vi "Automation Message Loop.vi"(8 "error in (no error)":errorcluster, 10 "Data Notifiers":T1, 11 "Message Queues":T2) -> (0 "error out":errorcluster)   [LabVIEW 2013, in "Automation.lvlib"]
uses:
  Automation.lvlib
  support/Message Queue/All Message Queues.ctl
  support/Message Queue/Message Cluster.ctl
  support/Data Notifiers/All Data Notifiers.ctl
  Acquisition/APD Notifier Cluster.ctl
  Piezo/Piezo display.ctl
  XY/XY Display.ctl
  Capacitive/Capacitive Signal Cluster.ctl
  Feedback/Error Signal.ctl
  Automation State.ctl
  Zscan Settings.ctl
  support/Message Queue/Enqueue Message (Single).vi
  <vilib>/Utility/error.llb/Error Cluster From Error Code.vi
  <vilib>/ErrorRing/Error Ring.xnode
  Piezo/Piezo.lvlib
  support/Message Queue/Message Queue.lvlib
  Acquisition/Acquisition.lvlib
  XY/XY.lvlib
  Capacitive/Capacitive.lvlib
  Feedback/Feedback.lvlib
  support/Data Notifiers/Data Notifiers.lvlib
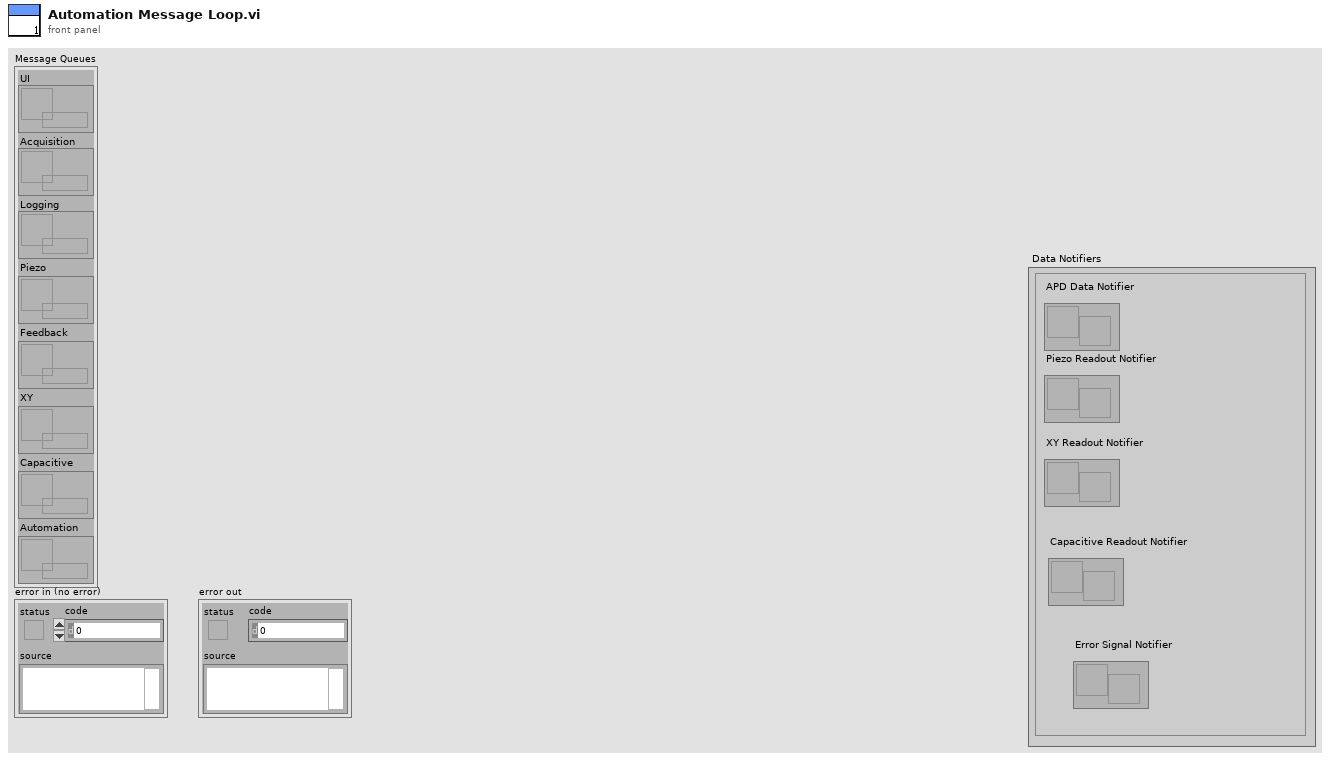
[diagram p1: front panel]
types:
  T1 = typedef "Data Notifiers.lvlib/All Data Notifiers.ctl" = cluster{"APD Data Notifier":refnum<notifier>, "Piezo Readout Notifier":refnum<notifier>, "XY Readout Notifier":refnum<notifier>, "Capacitive Readout Notifier":refnum<notifier>, "Error Signal Notifier":refnum<notifier>}
  T2 = typedef "Message Queue.lvlib/All Message Queues.ctl" = cluster{"UI":refnum<queue>, "Acquisition":refnum<queue>, "Logging":refnum<queue>, "Piezo":refnum<queue>, "Feedback":refnum<queue>, "XY":refnum<queue>, "Capacitive":refnum<queue>, "Automation":refnum<queue>}
  T3 = enum16{"Idle", "Waiting for lock", "Waiting for acquisition"}
  T4 = typedef "Automation.lvlib/Zscan Settings.ctl" = cluster{"Heights":dbl[], "Seconds per height":i32, "First Data Index":i32}
  T5 = typedef "Automation.lvlib/Automation State.ctl" = cluster{"State":enum16{"Idle", "Zscan"}, "Logging?":bool, "Zscan State":cluster{"State":enum16{"Idle", "Waiting for lock", "Waiting for acquisition"}, "ZScan Settings":T4, "Current Step":i32, "Current Cap Height":dbl, "Total Steps":i32, "Time Logging Started":dbl}}
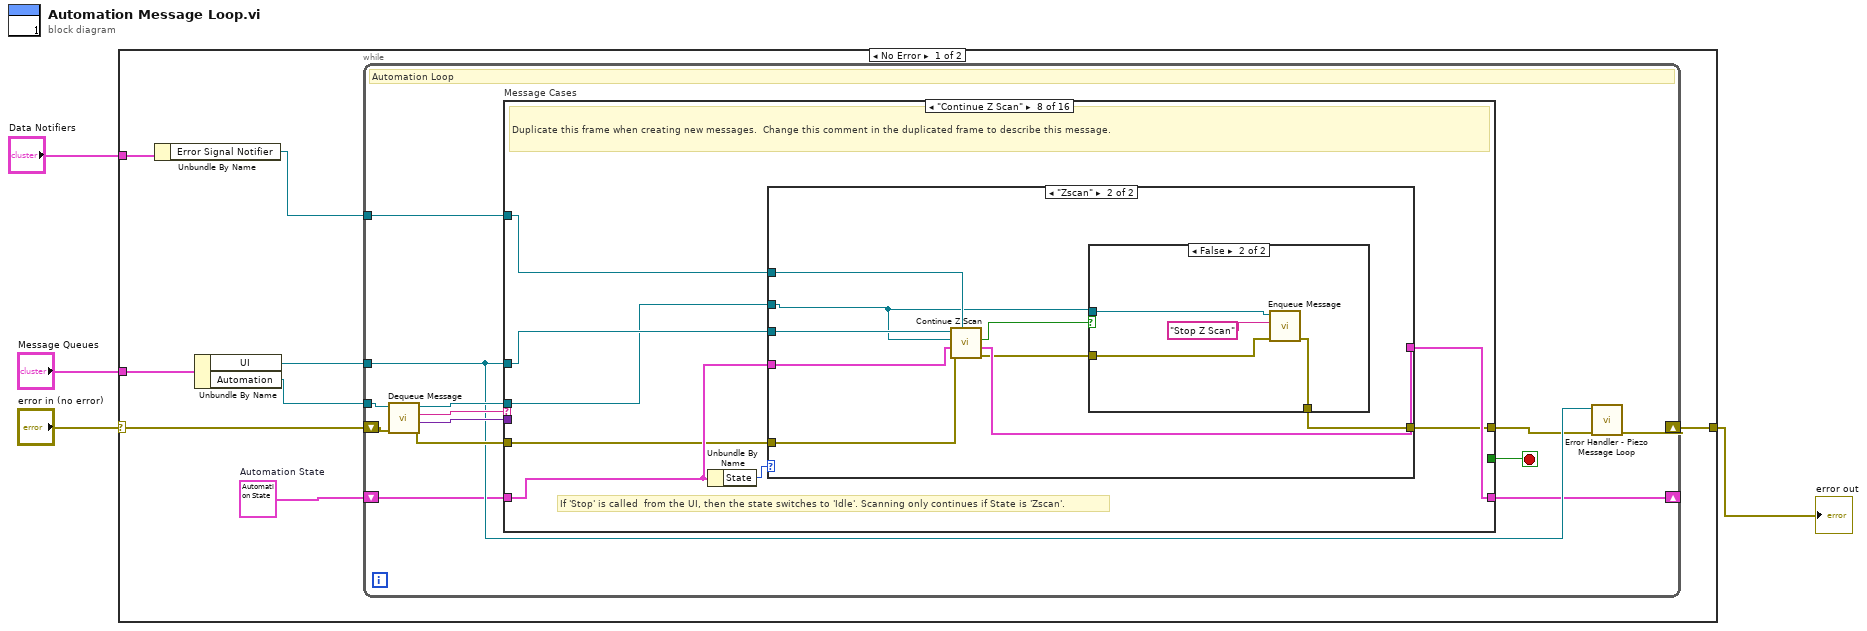
[diagram p0: block diagram]
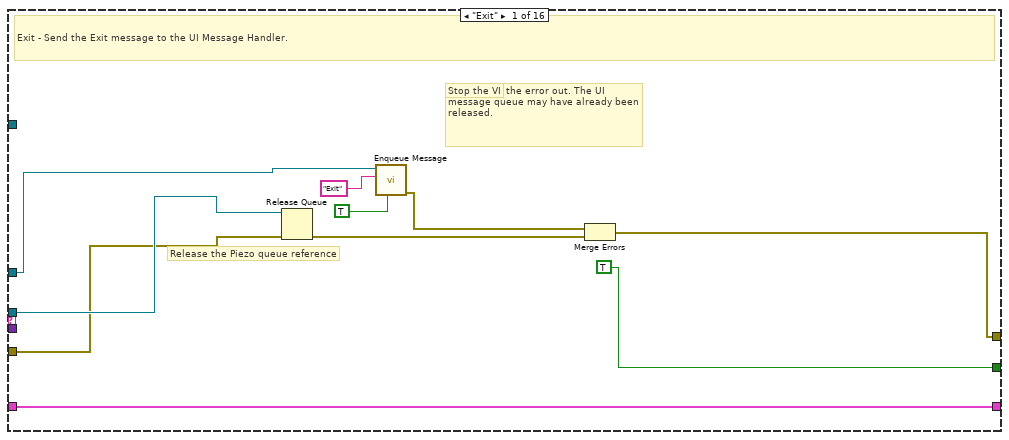
[diagram p2: hidden frame]
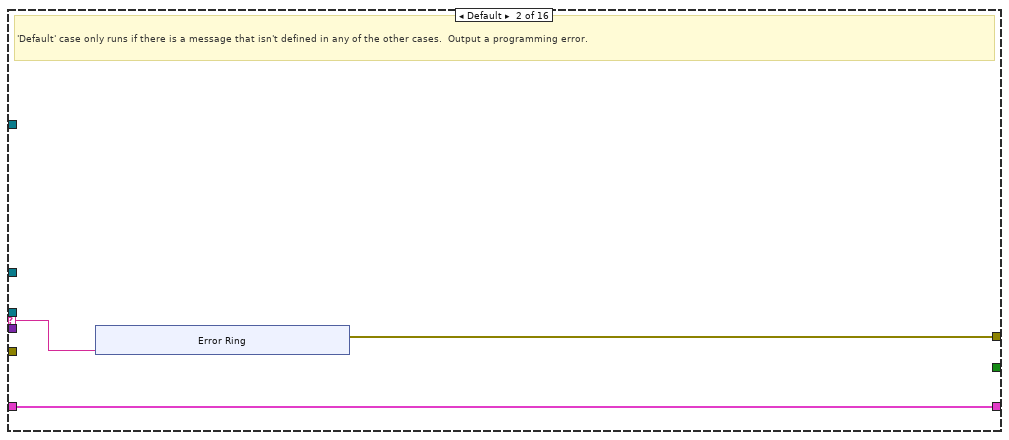
[diagram p3: hidden frame]
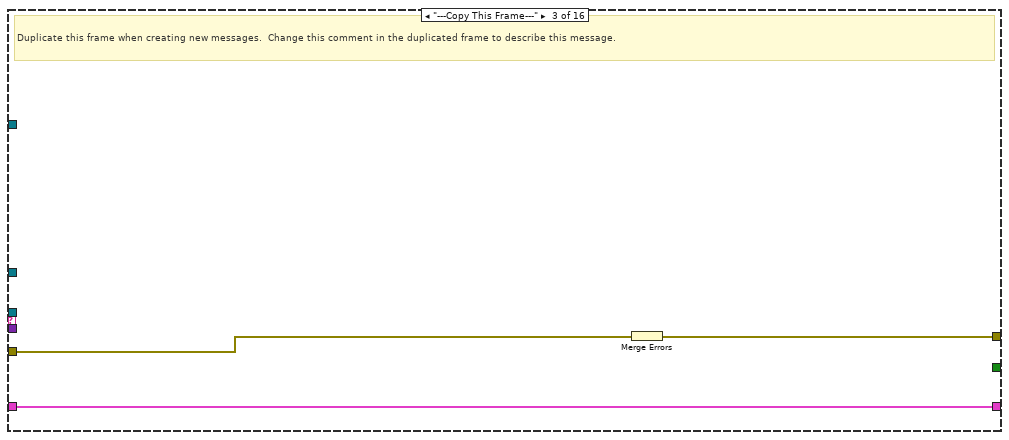
[diagram p4: hidden frame]
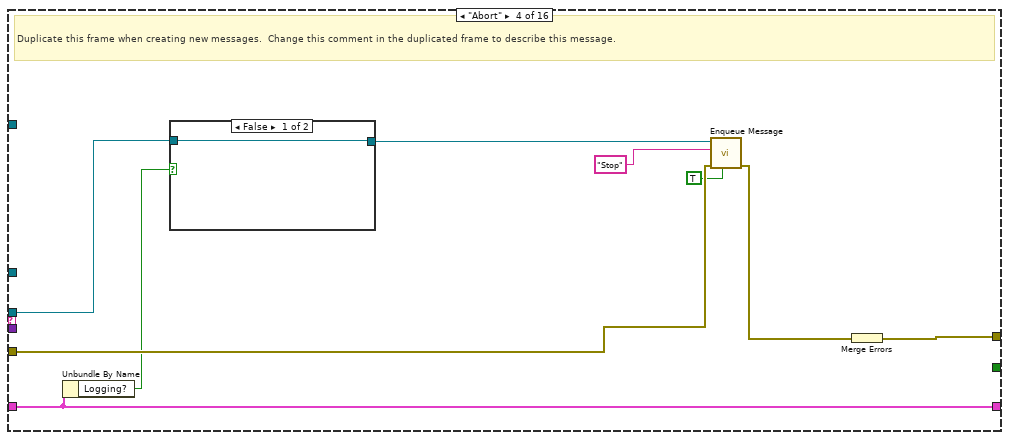
[diagram p5: hidden frame]
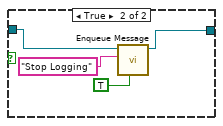
[diagram p6: hidden frame]
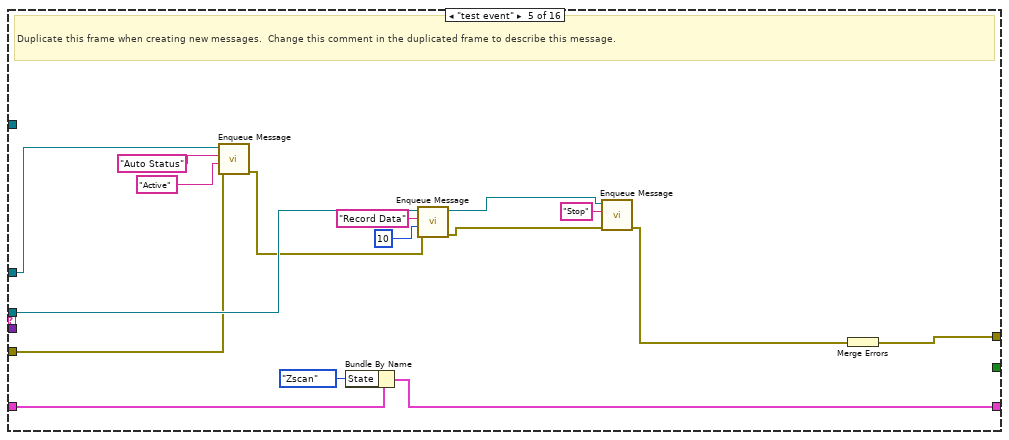
[diagram p7: hidden frame]
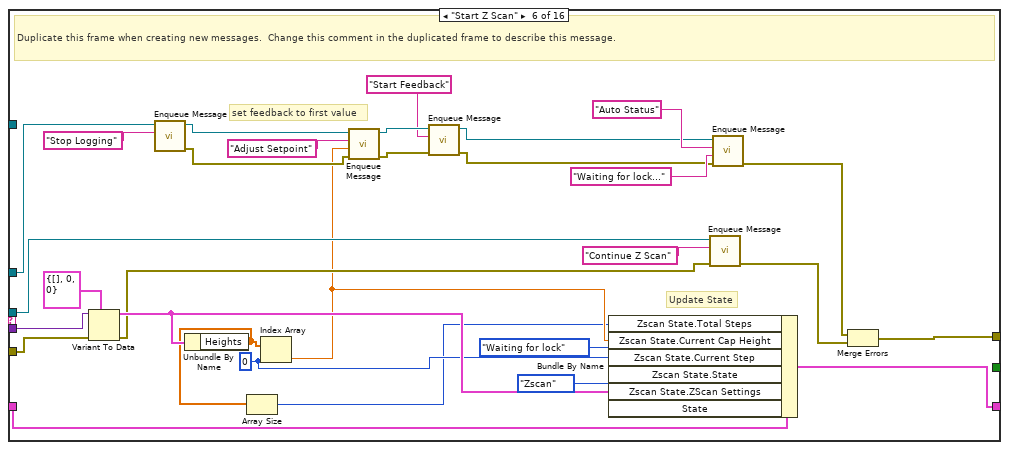
[diagram p8: hidden frame]
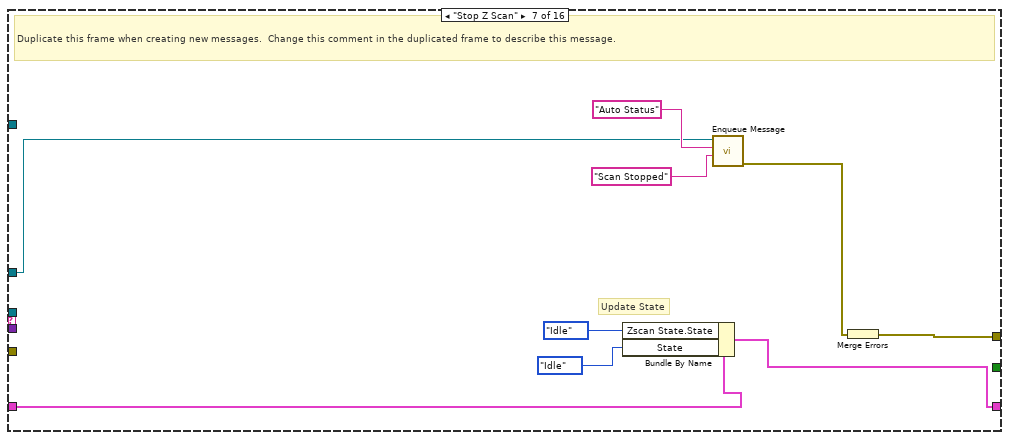
[diagram p9: hidden frame]
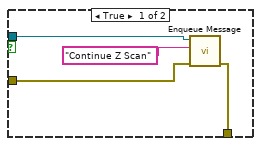
[diagram p11: hidden frame]
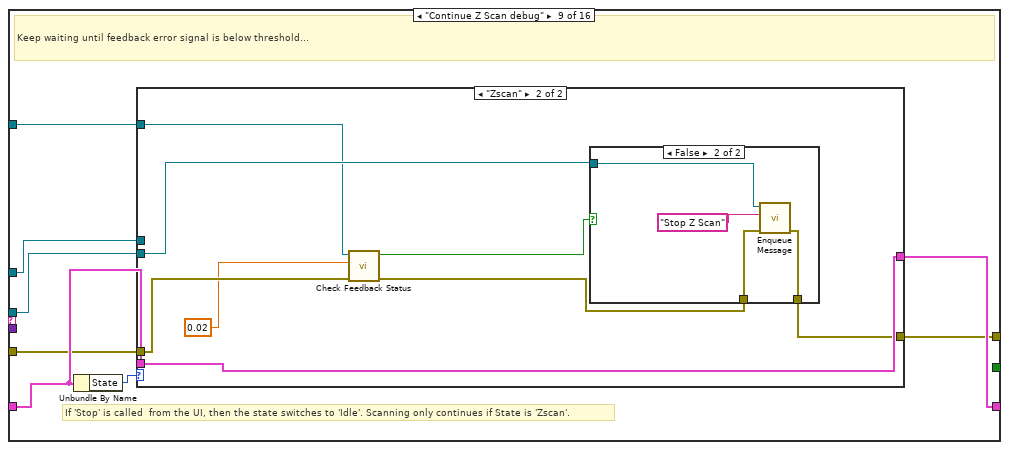
[diagram p12: hidden frame]
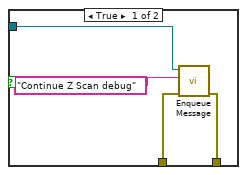
[diagram p14: hidden frame]
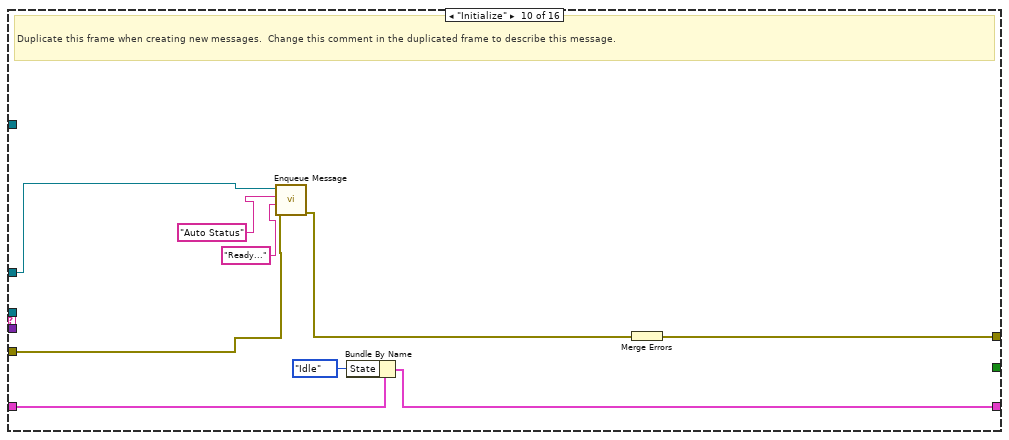
[diagram p15: hidden frame]
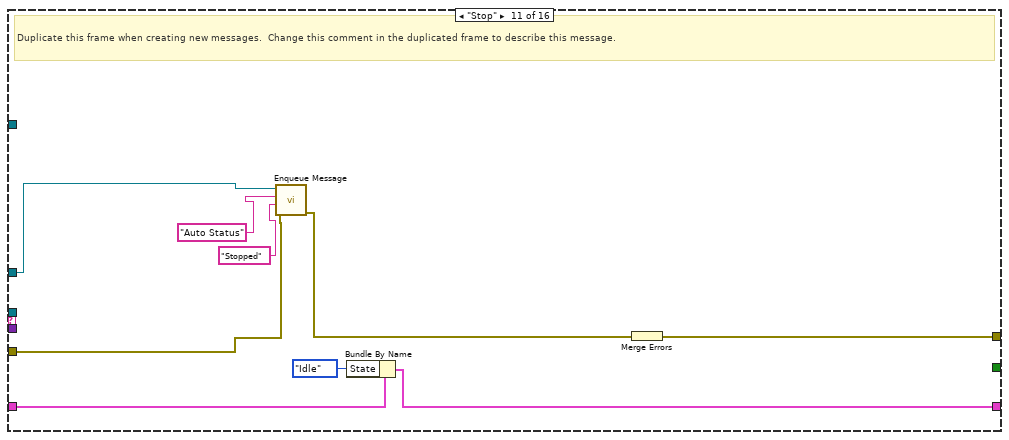
[diagram p16: hidden frame]
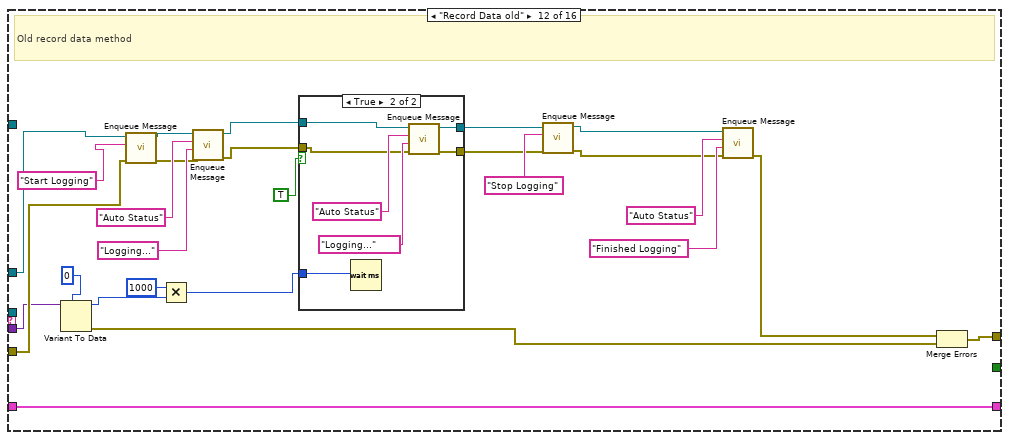
[diagram p17: hidden frame]
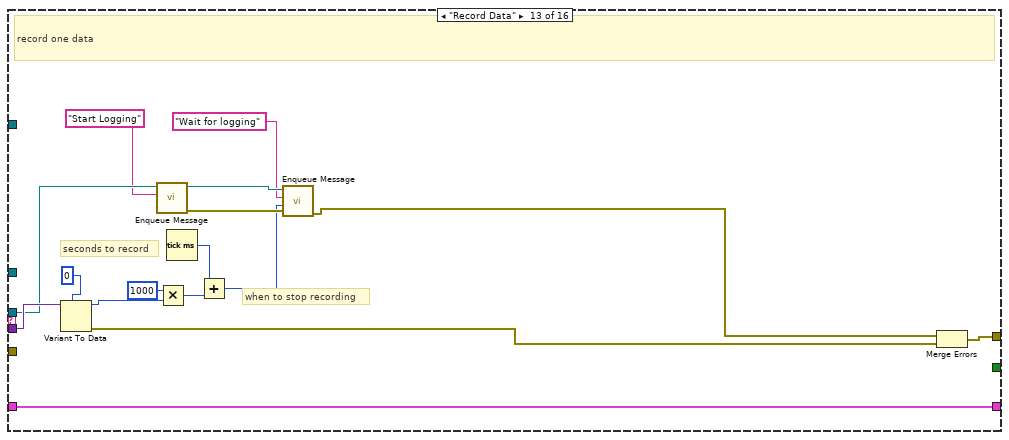
[diagram p19: hidden frame]
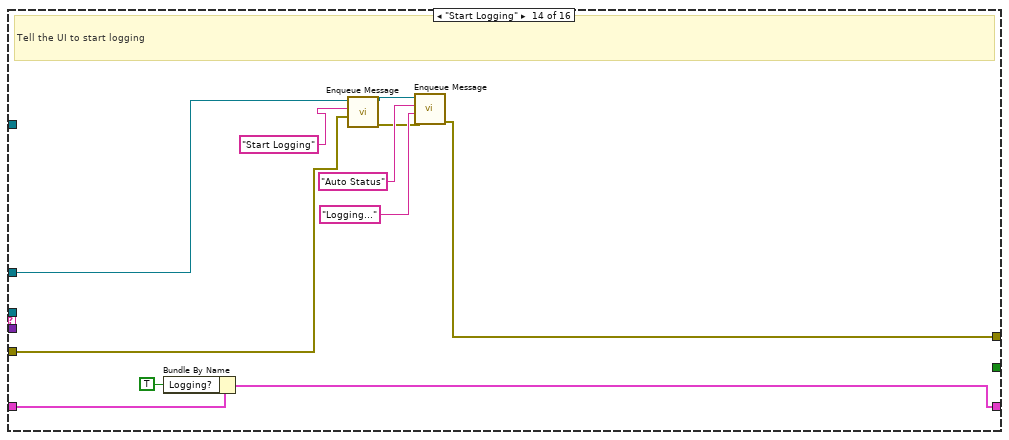
[diagram p20: hidden frame]
diagram:
  n1 = case shown="No Error" "error in (no error)" {
    selector: "error in (no error)" -> [w8 w284]
    tunnel: "Message Queues" -> [w12 _]
    tunnel: [w10 w284] -> w3
    tunnel: "Data Notifiers" -> [w6 _]
    frame No Error {
      w7 = T5 {"State"=enum."Idle", "Logging?"=FALSE, "Zscan State"={"State"=enum."Idle", "ZScan Settings"={"Heights"=[], "Seconds per height"=0, "First Data Index"=0}, "Current Step"=0, "Current Cap Height"=0.0, "Total Steps"=0, "Time Logging Started"=0.0}}  # Automation State
      n2 = Unbundle By Name(w6) -> ("Error Signal Notifier"=w5:refnum<notifier>)
      n3 = Unbundle By Name(w12) -> ("UI"=w9:refnum<queue>, "Automation"=w11:refnum<queue>)
      n4 = while {
        tunnel: w11 -> [w19]
        shift-right: [w17] -> w10
        shift-left: w8 -> [w24]
        tunnel: w9 -> [w18]
        shift-right: [w14] -> _
        shift-left: w7 -> [w15]
        tunnel: w5 -> [w13]
        stop <- w25 stop-if-true
        # "Automation Loop"
        n5 = call "Dequeue Message.vi"("error in (no error)"=w24, "Message Queue"=w19) -> ("error out"=w23:errorcluster, "Message Data"=w21:variant, "Message"=w22:string, "dup Message Queue"=w20:refnum<queue>)  [unwired: 6 in]
        n6 = case "Message Cases" shown="\"Continue Z Scan\"" w22 {
          selector: w22 -> [_ w38 _ _ _ _ _ _ _ _ _ _ _ _ _ _]
          tunnel: w20 -> [w30 _ _ w49 w77 w98 _ w123 w150 _ _ _ w234 _ _ w266]
          tunnel: w23 -> [w29 _ w48 w55 w70 w100 _ w119 w146 w172 w181 w201 _ w244 w254 w272]
          tunnel: [w28 w37 w47 w57 w78 w108 w117 w120 w147 w179 w188 w214 w239 w243 w256 w271] -> w16
          tunnel: [TRUE _ _ _ _ _ _ _ _ _ _ _ _ _ _ _] -> w25
          tunnel: w21 -> [_ _ _ _ _ w101 _ _ _ _ _ w194 w237 _ _ w273]
          tunnel: w18 -> [w31 _ _ _ w73 w95 w113 w124 w151 w176 w185 w212 _ w245 w255 _]
          tunnel: w15 -> [w26 w36 w46 w53 w65 w104 w110 w122 w149 w175 w184 w195 w238 w242 w252 w265]
          tunnel: [w26 w36 w46 w53 w66 w105 w109 w121 w148 w173 w182 w195 w238 w241 w251 w265] -> w14
          tunnel: w13 -> [_ _ _ _ _ _ _ w118 w145 _ _ _ _ _ _ _]
          frame "Exit" {
            # "Don't check the error out. The UI message queue may have already been released."
            # "Release the Piezo queue reference"
            # "Stop the VI"
            # "Exit - Send the Exit message to the UI Message Handler."
            n7 = Release Queue(queue=w30, error in (no error)=w29) -> (error out=w35:errorcluster)  [unwired: 1 in, 2 out]
            n8 = call-poly "Enqueue Message.vi"("Priority Message? (F)"=TRUE, "Message"="Exit", "Message Queue"=w31) -> ("error out"=w32:errorcluster)  [unwired: 7 in, 1 out]
            n9 = Merge Errors(w32, w35) -> (w28:errorcluster)
          }
          frame Default {
            # "'Default' case only runs if there is a message that isn't defined in any of the other cases.  Output a programming error."
            n10 = xnode "Error Ring"("parameter 0"=w38) -> ("error out"=w37:errorcluster)
          }
          frame "---Copy This Frame---" {
            # "Duplicate this frame when creating new messages.  Change this comment in the duplicated frame to describe this message."
            n11 = Merge Errors(w48) -> (w47:errorcluster)
          }
          frame "Abort" {
            # "Duplicate this frame when creating new messages.  Change this comment in the duplicated frame to describe this message."
            n12 = Unbundle By Name(w53) -> ("Logging?"=w52:bool)
            n13 = case shown="False" w52 {
              tunnel: w49 -> [w58 w61]
              tunnel: [w58 w60] -> w51
              frame False {
              }
              frame True {
                n14 = call-poly "Enqueue Message.vi"("Priority Message? (F)"=TRUE, "Message"="Stop Logging", "Message Queue"=w61) -> ("dup Message Queue"=w60:refnum<queue>)  [unwired: 7 in, 1 out]
              }
            }
            n15 = call-poly "Enqueue Message.vi"("Priority Message? (F)"=TRUE, "error in (no error)"=w55, "Message"="Stop", "Message Queue"=w51) -> ("error out"=w54:errorcluster)  [unwired: 6 in, 1 out]
            n16 = Merge Errors(w54) -> (w57:errorcluster)
          }
          frame "test event" {
            # "Duplicate this frame when creating new messages.  Change this comment in the duplicated frame to describe this message."
            n17 = call-poly "Enqueue Message.vi"("error in (no error)"=w70, "Message Data"="Active" ("Message"), "Message"="Auto Status", "Message Queue"=w73) -> ("error out"=w69:errorcluster)  [unwired: 6 in, 1 out]
            n18 = Bundle By Name(cluster=w65, "State"=enum16{"Idle", "Zscan"}."Zscan") -> (w66:T5)
            n19 = call-poly "Enqueue Message.vi"("error in (no error)"=w69, "Message Data"=u32 10 ("x"), "Message"="Record Data", "Message Queue"=w77) -> ("error out"=w68:errorcluster, "dup Message Queue"=w71:refnum<queue>)  [unwired: 6 in]
            n20 = call-poly "Enqueue Message.vi"("error in (no error)"=w68, "Message"="Stop", "Message Queue"=w71) -> ("error out"=w67:errorcluster)  [unwired: 7 in, 1 out]
            n21 = Merge Errors(w67) -> (w78:errorcluster)
          }
          frame "Start Z Scan" {
            w87 = 0 ("index")
            # "Update State"
            # "set feedback to first value"
            # "Duplicate this frame when creating new messages.  Change this comment in the duplicated frame to describe this message."
            n22 = Variant To Data(error in=w100, type=T4 {"Heights"=[], "Seconds per height"=0, "First Data Index"=0} ("ZScan Settings"), Variant=w101) -> (data=w92:T4, error out=w91:errorcluster)
            n23 = call-poly "Enqueue Message.vi"("Message"="Stop Logging", "Message Queue"=w95) -> ("error out"=w88:errorcluster, "dup Message Queue"=w93:refnum<queue>)  [unwired: 8 in]
            n24 = Unbundle By Name(w92) -> ("Heights"=w80:dbl[])
            n25 = Array Size(array=w80) -> (size(s)=w79:i32)
            n26 = Index Array(array=w80, index=w87) -> (element=w86:dbl)
            n27 = call-poly "Enqueue Message.vi"("error in (no error)"=w88, "Message Data"=w86, "Message"="Adjust Setpoint", "Message Queue"=w93) -> ("error out"=w82:errorcluster, "dup Message Queue"=w85:refnum<queue>)  [unwired: 6 in]
            n28 = call-poly "Enqueue Message.vi"("error in (no error)"=w82, "Message"="Start Feedback", "Message Queue"=w85) -> ("error out"=w83:errorcluster, "dup Message Queue"=w84:refnum<queue>)  [unwired: 7 in]
            n29 = Bundle By Name(cluster=w104, "Zscan State.Total Steps"=w79, "Zscan State.Current Cap Height"=w86, "Zscan State.Current Step"=w87, "Zscan State.State"=T3."Waiting for lock", "Zscan State.ZScan Settings"=w92, "State"=enum16{"Idle", "Zscan"}."Zscan") -> (w105:T5)
            n30 = call-poly "Enqueue Message.vi"("error in (no error)"=w91, "Message"="Continue Z Scan", "Message Queue"=w98) -> ("error out"=w90:errorcluster)  [unwired: 7 in, 1 out]
            n31 = call-poly "Enqueue Message.vi"("error in (no error)"=w83, "Message Data"="Waiting for lock..." ("Message"), "Message"="Auto Status", "Message Queue"=w84) -> ("error out"=w89:errorcluster)  [unwired: 6 in, 1 out]
            n32 = Merge Errors(w89, w90) -> (w108:errorcluster)
          }
          frame "Stop Z Scan" {
            # "Update State"
            # "Duplicate this frame when creating new messages.  Change this comment in the duplicated frame to describe this message."
            n33 = Bundle By Name(cluster=w110, "Zscan State.State"=T3."Idle", "State"=enum16{"Idle", "Zscan"}."Idle") -> (w109:T5)
            n34 = call-poly "Enqueue Message.vi"("Message Data"="Scan Stopped" ("Message"), "Message"="Auto Status", "Message Queue"=w113) -> ("error out"=w114:errorcluster)  [unwired: 7 in, 1 out]
            n35 = Merge Errors(w114) -> (w117:errorcluster)
          }
          frame "Continue Z Scan" {
            # "If 'Stop' is called  from the UI, then the state switches to 'Idle'. Scanning only continues if State is 'Zscan'."
            # "Duplicate this frame when creating new messages.  Change this comment in the duplicated frame to describe this message."
            n36 = Unbundle By Name(w122) -> ("State"=w125:enum16{"Idle", "Zscan"})
            n37 = case shown="\"Zscan\"" w125 {
              tunnel: w124 -> [_ w136]
              tunnel: w123 -> [_ w130]
              tunnel: w122 -> [w127 w135]
              tunnel: [w127 w134] -> w121
              tunnel: [w126 w128] -> w120
              tunnel: w119 -> [w126 w133]
              tunnel: w118 -> [_ w132]
              frame "Idle", Default {
              }
              frame "Zscan" {
                n38 = call "Continue Z Scan.vi"("Error Signal Notifier"=w132, "error in (no error)"=w133, "Automation State In"=w135, "Automation Queue"=w130, "UI Queue"=w136) -> ("error out"=w129:errorcluster, "Automation State Out"=w134:T5, "Keep looping?"=w131:bool)  [unwired: 4 in]
                n39 = case shown="False" w131 {
                  tunnel: w130 -> [w139 w143]
                  tunnel: w129 -> [w138 w142]
                  tunnel: [w137 w141] -> w128
                  frame True {
                    n40 = call-poly "Enqueue Message.vi"("error in (no error)"=w138, "Message"="Continue Z Scan", "Message Queue"=w139) -> ("error out"=w137:errorcluster)  [unwired: 7 in, 1 out]
                  }
                  frame False {
                    n41 = call-poly "Enqueue Message.vi"("error in (no error)"=w142, "Message"="Stop Z Scan", "Message Queue"=w143) -> ("error out"=w141:errorcluster)  [unwired: 7 in, 1 out]
                  }
                }
              }
            }
          }
          frame "Continue Z Scan debug" {
            # "If 'Stop' is called  from the UI, then the state switches to 'Idle'. Scanning only continues if State is 'Zscan'."
            # "Keep waiting until feedback error signal is below threshold..."
            n42 = Unbundle By Name(w149) -> ("State"=w152:enum16{"Idle", "Zscan"})
            n43 = case shown="\"Zscan\"" w152 {
              tunnel: w151 -> [_ _]
              tunnel: w150 -> [_ w162]
              tunnel: w149 -> [w154 w157]
              tunnel: [w154 w157] -> w148
              tunnel: [w153 w156] -> w147
              tunnel: w146 -> [w153 w160]
              tunnel: w145 -> [_ w161]
              frame "Idle", Default {
              }
              frame "Zscan" {
                n44 = call "Check Feedback Status.vi"("error in (no error)"=w160, "Threshold (um)"=0.02 ("x"), "Error Signal Notifier"=w161) -> ("error out"=w155:errorcluster, "Locked"=w158:bool)  [unwired: 7 in]
                n45 = case shown="False" w158 {
                  tunnel: w162 -> [w165 w169]
                  tunnel: [w164 w167] -> w156
                  tunnel: w155 -> [w163 w168]
                  frame True {
                    n46 = call-poly "Enqueue Message.vi"("error in (no error)"=w163, "Message"="Continue Z Scan debug", "Message Queue"=w165) -> ("error out"=w164:errorcluster)  [unwired: 7 in, 1 out]
                  }
                  frame False {
                    n47 = call-poly "Enqueue Message.vi"("error in (no error)"=w168, "Message"="Stop Z Scan", "Message Queue"=w169) -> ("error out"=w167:errorcluster)  [unwired: 7 in, 1 out]
                  }
                }
              }
            }
          }
          frame "Initialize" {
            # "Duplicate this frame when creating new messages.  Change this comment in the duplicated frame to describe this message."
            n48 = call-poly "Enqueue Message.vi"("error in (no error)"=w172, "Message Data"="Ready..." ("Message"), "Message"="Auto Status", "Message Queue"=w176) -> ("error out"=w171:errorcluster)  [unwired: 6 in, 1 out]
            n49 = Bundle By Name(cluster=w175, "State"=enum16{"Idle", "Zscan"}."Idle") -> (w173:T5)
            n50 = Merge Errors(w171) -> (w179:errorcluster)
          }
          frame "Stop" {
            # "Duplicate this frame when creating new messages.  Change this comment in the duplicated frame to describe this message."
            n51 = call-poly "Enqueue Message.vi"("error in (no error)"=w181, "Message Data"="Stopped" ("Message"), "Message"="Auto Status", "Message Queue"=w185) -> ("error out"=w180:errorcluster)  [unwired: 6 in, 1 out]
            n52 = Bundle By Name(cluster=w184, "State"=enum16{"Idle", "Zscan"}."Idle") -> (w182:T5)
            n53 = Merge Errors(w180) -> (w188:errorcluster)
          }
          frame "Record Data old" {
            # "Old record data method"
            n54 = Variant To Data(type=u32 0 ("milliseconds to wait"), Variant=w194) -> (data=w192:u32, error out=w189:errorcluster)  [unwired: 1 in]
            n55 = call-poly "Enqueue Message.vi"("error in (no error)"=w201, "Message"="Start Logging", "Message Queue"=w212) -> ("error out"=w200:errorcluster, "dup Message Queue"=w209:refnum<queue>)  [unwired: 7 in]
            n56 = Multiply(x=u32 1000, y=w192) -> (x*y=w190:u32)
            n57 = call-poly "Enqueue Message.vi"("error in (no error)"=w200, "Message Data"="Logging..." ("Message"), "Message"="Auto Status", "Message Queue"=w209) -> ("error out"=w199:errorcluster, "dup Message Queue"=w207:refnum<queue>)  [unwired: 6 in]
            n58 = case shown="True" TRUE {
              tunnel: w207 -> [w216 w223]
              tunnel: [w216 w220] -> w206
              tunnel: w199 -> [w215 w219]
              tunnel: [w215 w218] -> w198
              tunnel: w190 -> [_ w217]
              frame False {
              }
              frame True {
                n59 = Wait (ms)(milliseconds to wait=w217) -> ()  [unwired: 1 out]
                n60 = call-poly "Enqueue Message.vi"("error in (no error)"=w219, "Message Data"="Logging..." ("Message"), "Message"="Auto Status", "Message Queue"=w223) -> ("error out"=w218:errorcluster, "dup Message Queue"=w220:refnum<queue>)  [unwired: 6 in]
              }
            }
            n61 = call-poly "Enqueue Message.vi"("error in (no error)"=w198, "Message"="Stop Logging", "Message Queue"=w206) -> ("error out"=w197:errorcluster, "dup Message Queue"=w202:refnum<queue>)  [unwired: 7 in]
            n62 = call-poly "Enqueue Message.vi"("error in (no error)"=w197, "Message Data"="Finished Logging" ("Message"), "Message"="Auto Status", "Message Queue"=w202) -> ("error out"=w196:errorcluster)  [unwired: 6 in, 1 out]
            n63 = Merge Errors(w196, w189) -> (w214:errorcluster)
          }
          frame "Record Data" {
            # "when to stop recording"
            # "seconds to record"
            # "record one data"
            n64 = Variant To Data(type=u32 0 ("milliseconds to wait"), Variant=w237) -> (data=w228:u32, error out=w235:errorcluster)  [unwired: 1 in]
            n65 = call-poly "Enqueue Message.vi"("Message"="Start Logging", "Message Queue"=w234) -> ("error out"=w230:errorcluster, "dup Message Queue"=w233:refnum<queue>)  [unwired: 8 in]
            n66 = Multiply(x=u32 1000, y=w228) -> (x*y=w226:u32)
            n67 = Tick Count (ms)() -> (millisecond timer value=w225:u32)
            n68 = Add(x=w225, y=w226) -> (x+y=w224:u32)
            n69 = call-poly "Enqueue Message.vi"("error in (no error)"=w230, "Message Data"=w224, "Message"="Wait for logging", "Message Queue"=w233) -> ("error out"=w229:errorcluster)  [unwired: 6 in, 1 out]
            n70 = Merge Errors(w229, w235) -> (w239:errorcluster)
          }
          frame "Start Logging" {
            # "Tell the UI to start logging"
            n71 = Bundle By Name(cluster=w242, "Logging?"=TRUE) -> (w241:T5)
            n72 = call-poly "Enqueue Message.vi"("Message Data"=w244, "Message"="Start Logging", "Message Queue"=w245) -> ("error out"=w246:errorcluster, "dup Message Queue"=w247:refnum<queue>)  [unwired: 7 in]
            n73 = call-poly "Enqueue Message.vi"("error in (no error)"=w246, "Message Data"="Logging..." ("Message"), "Message"="Auto Status", "Message Queue"=w247) -> ("error out"=w243:errorcluster)  [unwired: 6 in, 1 out]
          }
          frame "Stop Logging" {
            # "Tell the UI to start logging"
            n74 = call-poly "Enqueue Message.vi"("error in (no error)"=w254, "Message"="Stop Logging", "Message Queue"=w255) -> ("error out"=w257:errorcluster, "dup Message Queue"=w258:refnum<queue>)  [unwired: 7 in]
            n75 = Bundle By Name(cluster=w252, "Logging?"=FALSE) -> (w251:T5)
            n76 = call-poly "Enqueue Message.vi"("error in (no error)"=w257, "Message Data"="Finished Logging" ("Message"), "Message"="Auto Status", "Message Queue"=w258) -> ("error out"=w256:errorcluster)  [unwired: 6 in, 1 out]
          }
          frame "Wait for logging" {
            # "time remaining"
            # "Tell the UI to start logging"
            n77 = Variant To Data(type=u32 0 ("milliseconds to wait"), Variant=w273) -> (data=w267:u32)  [unwired: 1 in, 1 out]
            n78 = Tick Count (ms)() -> (millisecond timer value=w270:u32)
            n79 = Subtract(x=w270, y=w267) -> (x-y=w269:u32)
            n80 = Unbundle By Name(w265) -> ("Logging?"=w264:bool)
            n81 = Greater?(x=w269, y=u32 0) -> (0:w263:bool)
            n82 = And(x=w263, y=w264) -> (x .and. y?=w262:bool)
            n83 = case shown="True" w262 {
              tunnel: w266 -> [w277 w283]
              tunnel: w272 -> [w276 w281]
              tunnel: [w275 w280] -> w271
              tunnel: w267 -> [_ w279]
              frame False {
                n84 = call-poly "Enqueue Message.vi"("error in (no error)"=w276, "Message"="Stop Logging", "Message Queue"=w277) -> ("error out"=w275:errorcluster)  [unwired: 7 in, 1 out]
              }
              frame True {
                # "keep waiting..."
                n85 = call-poly "Enqueue Message.vi"("error in (no error)"=w281, "Message Data"=w279, "Message"="Wait for logging", "Message Queue"=w283) -> ("error out"=w280:errorcluster)  [unwired: 6 in, 1 out]
              }
            }
          }
        }
        n86 = call "Error Handler - Piezo Message Loop.vi"("error in (no error)"=w16, "Message Queue"=w18) -> ("dup error in"=w17:errorcluster)  [unwired: 8 in, 1 out]
      }
    }
    frame Error {
    }
  }
  "error out" <- w3
